vi "To String.vi"(8 "error in (no error)":errorcluster, 11 "JSON Null in":refnum<class "JSON Null.lvclass">) -> (0 "error out":errorcluster, 3 "String":string)   [LabVIEW 2017, in "LVJSON.lvlib" / "JSON Null.lvclass"]
uses:
  JSON Null.lvclass
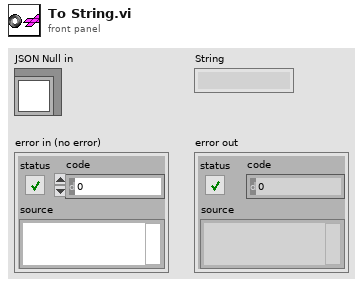
[diagram p1: front panel]
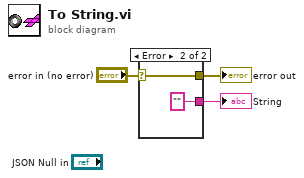
[diagram p0: block diagram]
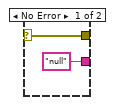
[diagram p2: hidden frame]
diagram:
  n1 = case shown="Error" "error in (no error)" {
    selector: "error in (no error)" -> [w4 w7]
    tunnel: ["null" ("String") "" ("String")] -> w3
    tunnel: [w4 w7] -> w1
    frame No Error {
    }
    frame Error {
    }
  }
  "String" <- w3
  "error out" <- w1
